vi "FRS.vi"(0 "System no.":i32=1 min=1 max=4 step=1, 2 "Routines to start":string[](array[string]), 5 "error in":errorcluster) -> (19 "error out":errorcluster)   [LabVIEW 2026]
doc: "Starts the given fast alignment routine (one or more). Routine must be predefined, e.g. with FDR or FDG. \n\nC-887, E-712, E-727.AS:"
panel:
  # "Starts the given fast alignment procedure (one or more). Procedure \nmust be predefined, e.g. with FDR or FDG."
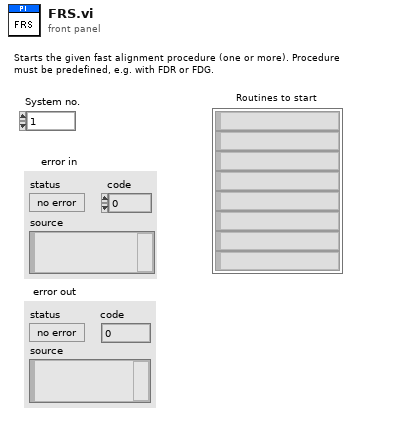
[diagram p1: front panel]
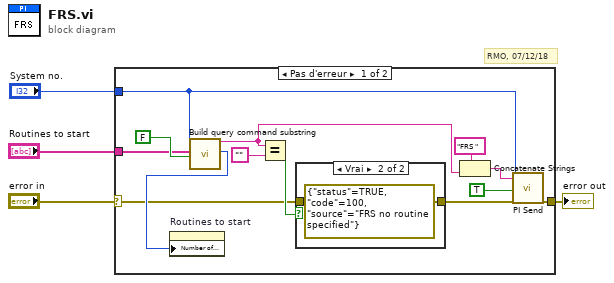
[diagram p0: block diagram]
diagram:
  # "RMO, 07/12/18"
  n1 = case shown="Pas d'erreur" "error in" {
    selector: "error in" -> [w5 w20]
    tunnel: "Routines to start" -> [w8 _]
    tunnel: [w6 w20] -> w3
    tunnel: "System no." -> [w11 _]
    frame No Error {
      n2 = call "Build query command substring.vi"("System no."=w11, "Axes to query in"=w8, "Query\nAll axes?"=FALSE ("Query\nAll axes?")) -> ("Command substring"=w13:string, "Number of rows"=w12:u32)  [unwired: 3 in, 12 out]
      n3 = property on="Routines to start" class="Tabl (strict)"("Number of Rows"=w12) -> ()  [unwired: 2 in, 2 out]
      n4 = Equal?(x=w13, y="" ("x")) -> (x = y?=w9:bool)
      n5 = case shown="Vrai" w9 {
        tunnel: [w18 errorcluster {"status"=TRUE, "code"=100, "source"="FRS no routine specified"} ("error out")] -> w7
        tunnel: w5 -> [w18 _]
        frame False {
        }
        frame True {
        }
      }
      n6 = Concatenate Strings("FRS ", w13) -> (w15:string)
      n7 = call "PI Send.vi"("System no."=w11, "String to send"=w15, "Attach termination char.?"=TRUE ("Attach Linefeed?"), "error in"=w7) -> ("error out"=w6:errorcluster)  [unwired: 2 in, 13 out]
    }
    frame Error {
    }
  }
  "error out" <- w3
